vi "movemotor.vi"(2 "error in (no error)":errorcluster caption="错误输入（无错误）", 3 "target pos":dbl, 4 "OneMotion 输入":refnum<class "OneMotion.lvclass">) -> (0 "error out":errorcluster caption="错误输出", 1 "OneMotion 输出":refnum<class "OneMotion.lvclass">)   [LabVIEW 2016, in "MotionControl_UFO_3DOF.lvlib" / "OneMotion.lvclass"]
uses:
  <userlib>/MotionControl_UFO_3DOF/OneMotion/OneMotion.lvclass
  <userlib>/MotionControl_UFO_3DOF/OneMotion/hard limit option.ctl
  <userlib>/MotionControl_UFO_3DOF/OneMotion/OneMotion.lvclass/OneMotion.ctl
  <userlib>/MotionControl_UFO_3DOF/StepMotor/BasicMovPara.ctl
  <userlib>/MotionControl_UFO_3DOF/StepMotor/StepMotor.lvclass/StepMotor.ctl
  <userlib>/MotionControl_UFO_3DOF/StepMotor/StepMotor.lvclass
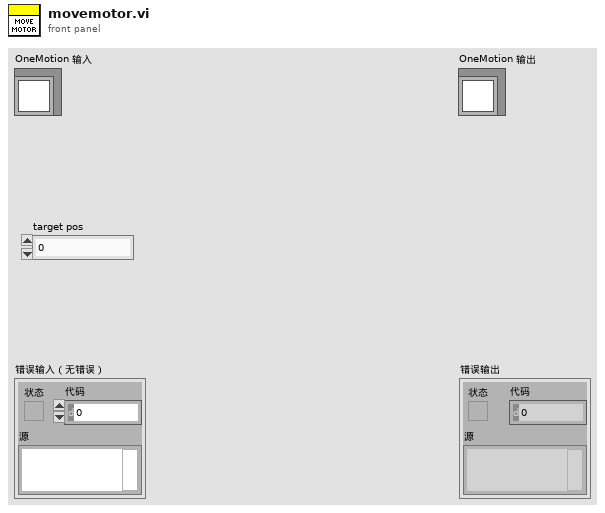
[diagram p1: front panel]
types:
  T1 = typedef "MotionControl_UFO_3DOF.lvlib/OneMotion.lvclass/hard limit option.ctl" = enum16{"STOP, and a 0.5s timeout constraint in move", "STOP, and move disabled"}
  T2 = typedef "MotionControl_UFO_3DOF.lvlib/StepMotor.lvclass/BasicMovPara.ctl" = cluster{"speed":i32, "POS / QEC":i32, "timeout":i32}
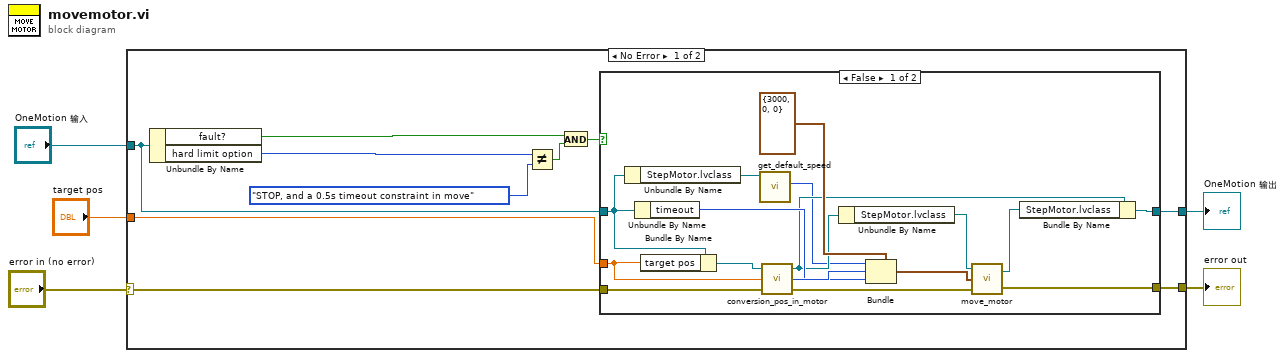
[diagram p0: block diagram]
diagram:
  n1 = case shown="No Error" "error in (no error)" {
    selector: "error in (no error)" -> [w15 w35]
    tunnel: [w14 w35] -> w4
    tunnel: [w12 w34] -> w2
    tunnel: "OneMotion 输入" -> [w11 w34]
    tunnel: "target pos" -> [w13 _]
    frame No Error {
      n2 = Unbundle By Name(w11) -> ("fault?"=w8:bool, "hard limit option"=w10:T1)
      n3 = Not Equal?(x=w10, y=hard_limit_option."STOP, and a 0.5s timeout constraint in move" ("hard limit option")) -> (x != y?=w6:bool)
      n4 = And(x=w8, y=w6) -> (x .and. y?=w7:bool)
      n5 = case shown="False" w7 {
        tunnel: w15 -> [w31 w32]
        tunnel: [w18 w32] -> w14
        tunnel: w13 -> [w25 _]
        tunnel: [w21 w33] -> w12
        tunnel: w11 -> [w20 w33]
        frame False {
          n6 = Unbundle By Name(w20) -> ("StepMotor.lvclass"=w17:refnum<class "StepMotor.lvclass">)
          n7 = Unbundle By Name(w20) -> ("timeout"=w27:u32)
          n8 = Bundle By Name(cluster=w20, "target pos"=w25) -> (w22:refnum<class "OneMotion.lvclass">)
          n9 = call <userlib>:"get_default_speed.vi"("StepMotor输入"=w17) -> ("expected speed"=w16:i32)  [unwired: 8 in, 2 out]
          n10 = call <userlib>:"conversion_pos_in_motor.vi"("error in (no error)"=w31, "pos"=w25, "OneMotion 输入"=w22) -> ("error out"=w30:errorcluster, "pos in motor"=w28:i32, "OneMotion 输出"=w23:refnum<class "OneMotion.lvclass">)
          n11 = Unbundle By Name(w23) -> ("StepMotor.lvclass"=w24:refnum<class "StepMotor.lvclass">)
          n12 = Bundle(cluster=T2 {"speed"=3000, "POS / QEC"=0, "timeout"=0} ("Basic Move Parameters"), "speed"=w16, "POS / QEC"=w28, "timeout"=w27) -> (w26:T2)
          n13 = call-dynamic "move_motor.vi"("error in (no error)"=w30, "Basic Move Parameters"=w26, "StepMotor输入"=w24) -> ("error out"=w18:errorcluster, "StepMotor输出"=w19:refnum<class "StepMotor.lvclass">)
          n14 = Bundle By Name(cluster=w23, "StepMotor.lvclass"=w19) -> (w21:refnum<class "OneMotion.lvclass">)
        }
        frame True {
        }
      }
    }
    frame Error {
    }
  }
  "error out" <- w4
  "OneMotion 输出" <- w2
